vi "HH Command Disable.vi"(11 "_Command":refnum<vi>) -> ()   [LabVIEW 2016]
uses:
  <vilib>/Powertrain Controls/Device Drivers/DCM/HH/RT/Setup.ctl
  <vilib>/Powertrain Controls/Device Drivers/DCM/HH/FPGA/Mode.ctl
  <vilib>/Powertrain Controls/Device Drivers/DCM/Rev0/FPGA/Digital Channel.ctl
  <vilib>/Powertrain Controls/Device Drivers/DCM/HH/RT/Angle Control.ctl
  <vilib>/Powertrain Controls/Device Drivers/DCM/HH/RT/DCM - RT - HH.lvlib
  <vilib>/Powertrain Controls/Device Drivers/DCM/HH/FPGA/DCM - FPGA - HH.lvlib
  <vilib>/Powertrain Controls/Device Drivers/DCM/Rev0/FPGA/DCM - FPGA.lvlib
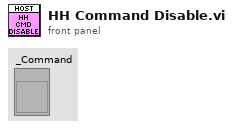
[diagram p1: front panel]
types:
  T1 = typedef "DCM - RT - HH.lvlib/Setup.ctl" = cluster{"Mode":T2, "Digital Input":T3, "Polarity":bool, "Frequency [Hz]":sgl, "Duty Cycle [%]":sgl, "TDC Offset [CAD]":sgl, "Window Start [DBTDC]":sgl, "Window End [DBTDC]":sgl, "Angles":T4[], "Skip Fire":bool, "Skip Fire Index":u8}
  T2 = typedef "DCM - FPGA - HH.lvlib/Mode.ctl" = enum8{"Off", "Direct", "Pulse Width Modulation", "Engine Position Tracking"}
  T3 = typedef "DCM - FPGA.lvlib/Digital Channel.ctl" = enum8{"Unused", "User OS", "Diff IO 1", "Diff IO 2", "Diff IO 3", "Diff IO 4", "Diff IO 5", "Diff IO 6", "Diff IO 7", "Diff IO 8", "Aux 1", "Aux 2", "Aux 3", "Aux 4", "Aux 5", "Aux 6", "Aux 7", "Aux 8", "Aux 9", "Aux 10", "Aux 11", "Aux 12", "Aux 13", "Aux 14", "Aux 15", "Aux 16"}
  T4 = typedef "DCM - RT - HH.lvlib/Angle Control.ctl" = cluster{"Enable":bool, "Location [DBTDC]":sgl, "Duration [s]":sgl}
  T5 = enum8{"Enabled", "Disabled", "Disabled and Grayed Out"}[]
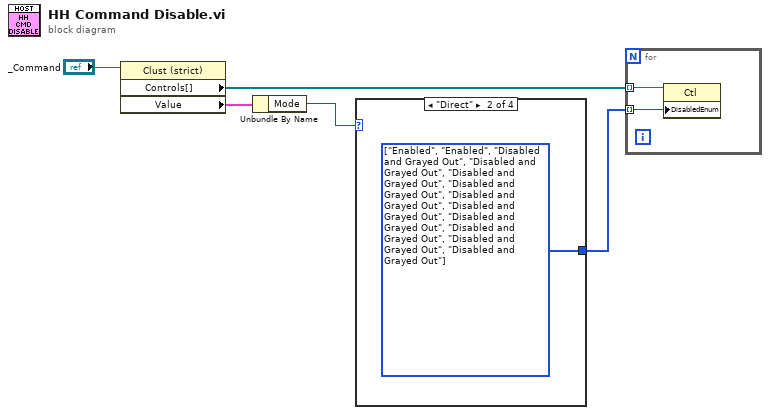
[diagram p0: block diagram]
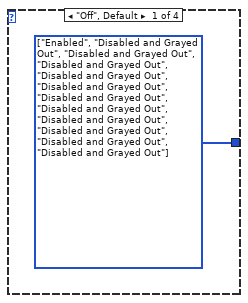
[diagram p2: hidden frame]
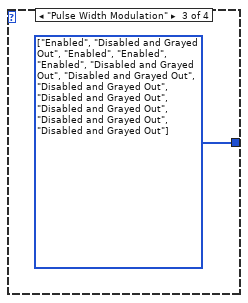
[diagram p3: hidden frame]
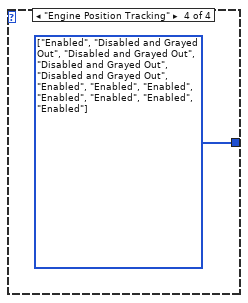
[diagram p4: hidden frame]
diagram:
  n1 = property class="Clust (strict)"(reference="_Command") -> ("Controls[]"=w2:refnum<vi>[], "Value"=w1:T1)  [unwired: 1 in, 2 out]
  n2 = Unbundle By Name(w1) -> ("Mode"=w4:T2)
  n3 = case shown="\"Direct\"" w4 {
    tunnel: [w6 w7 w8 w9] -> w3
    frame "Off", Default {
      w6 = T5 [enum."Enabled", enum."Disabled and Grayed Out", enum."Disabled and Grayed Out", enum."Disabled and Grayed Out", enum."Disabled and Grayed Out", enum."Disabled and Grayed Out", enum."Disabled and Grayed Out", enum."Disabled and Grayed Out", enum."Disabled and Grayed Out", enum."Disabled and Grayed Out", enum."Disabled and Grayed Out", enum."Disabled and Grayed Out"] items=["Enabled", "Disabled", "Disabled and Grayed Out"]
    }
    frame "Direct" {
      w7 = T5 [enum."Enabled", enum."Enabled", enum."Disabled and Grayed Out", enum."Disabled and Grayed Out", enum."Disabled and Grayed Out", enum."Disabled and Grayed Out", enum."Disabled and Grayed Out", enum."Disabled and Grayed Out", enum."Disabled and Grayed Out", enum."Disabled and Grayed Out", enum."Disabled and Grayed Out", enum."Disabled and Grayed Out"] items=["Enabled", "Disabled", "Disabled and Grayed Out"]
    }
    frame "Pulse Width Modulation" {
      w8 = T5 [enum."Enabled", enum."Disabled and Grayed Out", enum."Enabled", enum."Enabled", enum."Enabled", enum."Disabled and Grayed Out", enum."Disabled and Grayed Out", enum."Disabled and Grayed Out", enum."Disabled and Grayed Out", enum."Disabled and Grayed Out", enum."Disabled and Grayed Out", enum."Disabled and Grayed Out"] items=["Enabled", "Disabled", "Disabled and Grayed Out"]
    }
    frame "Engine Position Tracking" {
      w9 = T5 [enum."Enabled", enum."Disabled and Grayed Out", enum."Disabled and Grayed Out", enum."Disabled and Grayed Out", enum."Disabled and Grayed Out", enum."Enabled", enum."Enabled", enum."Enabled", enum."Enabled", enum."Enabled", enum."Enabled", enum."Enabled"] items=["Enabled", "Disabled", "Disabled and Grayed Out"]
    }
  }
  n4 = for {
    tunnel: w3 -> [w10] mode=indexing
    tunnel: w2 -> [w11] mode=indexing
    n5 = property class="Ctl"(reference=w11, "DisabledEnum"=w10) -> ()  [unwired: 1 in, 2 out]
  }
